vi "Filterout.vi"(9 "elements":i32[](array[numeric]), 11 "Array":dbl[](array[numeric])) -> (3 "output":dbl[](array[numeric]))   [LabVIEW 2014]
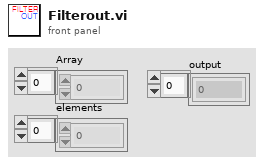
[diagram p1: front panel]
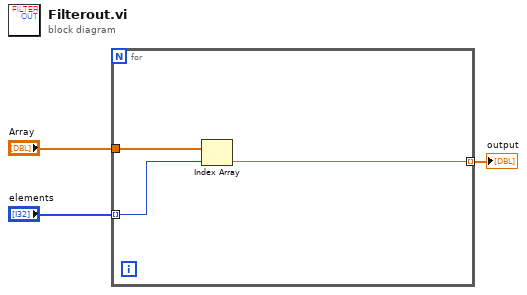
[diagram p0: block diagram]
diagram:
  n1 = for {
    tunnel: "elements" -> [w5] mode=indexing
    tunnel: "Array" -> [w6]
    tunnel: [w4] -> w1 mode=indexing
    n2 = Index Array(array=w6, index=w5) -> (element=w4:dbl)
  }
  "output" <- w1
